vi "test_ClientFGV_GetClient_ClientCreated.vi"(8 "error in":errorcluster) -> (0 "error out":errorcluster, 2 "result":string, 3 "pass":bool)   [LabVIEW 2020, in "MeasurementServerTests.lvlib" / "gRPC Utilities Tests.lvlib"]
uses:
  gRPC Utilities Tests.lvlib
  Runtime/MeasurementLink gRPC Utilities/gRPC Client Pool Helpers/Action.ctl
  Runtime/MeasurementLink gRPC Utilities/MeasurementLink gRPC Utilities.lvlib
  <vilib>/gRPC/LabVIEW gRPC Library/Shared/grpcId.ctl
  <vilib>/gRPC/LabVIEW gRPC Library/grpc-lvsupport-release.lvlib
  Action.ctl
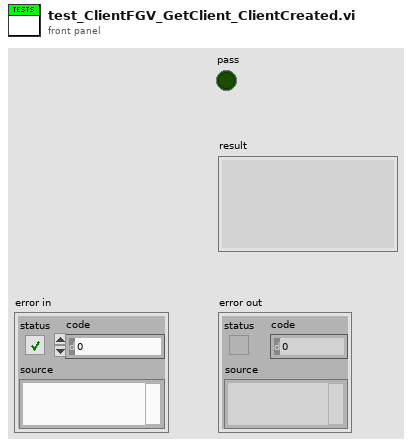
[diagram p1: front panel]
types:
  T1 = typedef "Action.ctl" = enum16{"Increment Id", "Reset", "Error on Next Call"}
  T2 = typedef "grpc-lvsupport-release.lvlib/grpcId.ctl" = u64
  T3 = typedef "MeasurementLink gRPC Utilities.lvlib/Action.ctl" = enum16{"Get Client", "Recreate Client"}
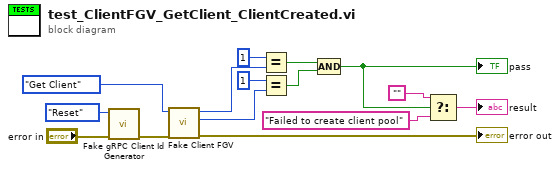
[diagram p0: block diagram]
diagram:
  n1 = call "Fake gRPC Client Id Generator.vi"("error in"="error in", "action"=Action."Reset") -> ("error out"=w4:errorcluster)  [unwired: 8 in, 1 out]
  n2 = call "Fake Client FGV.vi"("error in"=w4, "action"=Action."Get Client") -> ("error out"=→"error out":errorcluster, "unique id out"=w10:u64, "grpc client id"=w14:T2)  [unwired: 7 in]
  n3 = Equal?(x=T2 1, y=w14) -> (x = y?=w13:bool)
  n4 = Equal?(x=u64 1, y=w10) -> (x = y?=w12:bool)
  n5 = Compound Arithmetic op=AND(w13, w12) -> (w9:bool)
  "pass" <- w9
  n6 = Select(t="", s=w9, f="Failed to create client pool") -> (s? t:f=→"result":string)
